vi "MultiplyMatrixRows.vi"(1 "Column":string[](array[string]), 2 "Row":string[](array[string])) -> (0 "Output":string)   [LabVIEW 2011]
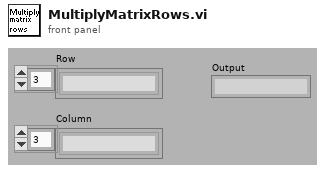
[diagram p1: front panel]
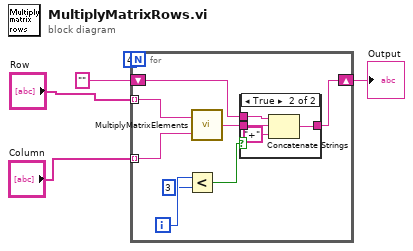
[diagram p0: block diagram]
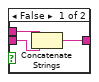
[diagram p2: hidden frame]
diagram:
  n1 = for {
    N: 4 -> [_]
    tunnel: "Row" -> [w13] mode=indexing
    tunnel: "Column" -> [w12] mode=indexing
    shift-right: [w6] -> w1
    shift-left: "" -> [w10]
    i -> [w9]
    n2 = Less?(x=w9, y=3) -> (x < y?=w7:bool)
    n3 = call "MultiplyMatrixElements.vi"("Element2"=w12, "Element1"=w13) -> ("Element Out"=w11:string)
    n4 = case shown="True" w7 {
      tunnel: w11 -> [w15 w20]
      tunnel: w10 -> [w16 w19]
      tunnel: [w14 w18] -> w6
      frame False {
        n5 = Concatenate Strings(w16, w15) -> (w14:string)
      }
      frame True {
        n6 = Concatenate Strings(w19, w20, "+" ("string")) -> (w18:string)
      }
    }
  }
  "Output" <- w1
